vi "Initialize.vi"(8 "error in (no error)":errorcluster, 10 "CommandText":string, 11 "PathCommands.ClosePath in":refnum<class "PathCommands.ClosePath.lvclass">) -> (0 "error out":errorcluster, 3 "PathCommands.ClosePath out":refnum<class "PathCommands.ClosePath.lvclass">)   [LabVIEW 2019, in "PathCommands.ClosePath.lvclass"]
uses:
  PathCommands.ClosePath.lvclass
  PathCommands/PathCommands.lvclass
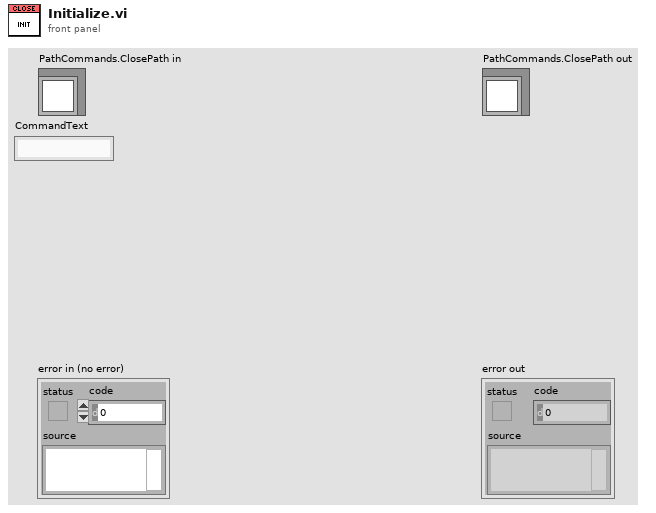
[diagram p1: front panel]
types:
  T1 = enum16{"None", "After", "Before", "Last", "First"}[]
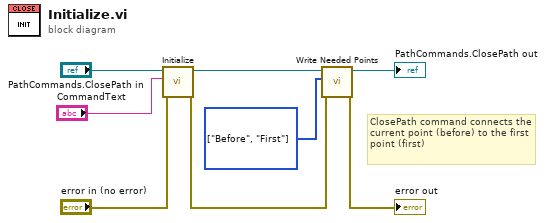
[diagram p0: block diagram]
diagram:
  w3 = T1 [enum."Before", enum."First"] items=["None", "After", "Before", "Last", "First"] ("Needed Points")
  # "ClosePath command connects the current point (before) to the first point (first)"
  n1 = call-parent "Initialize.vi"("error in (no error)"="error in (no error)", "CommandText"="CommandText", "PathCommands in"="PathCommands.ClosePath in") -> ("error out"=w2:errorcluster, "PathCommands out"=w5:refnum<class "PathCommands.ClosePath.lvclass">)  [unwired: 7 in]
  n2 = call-dynamic "Write Needed Points.vi"("error in (no error)"=w2, "Needed Points"=w3, "PathCommands in"=w5) -> ("error out"=→"error out":errorcluster, "PathCommands out"=→"PathCommands.ClosePath out":refnum<class "PathCommands.ClosePath.lvclass">)  [unwired: 7 in]
